vi "Cell Alignment to Horizontal and Vertical.vi"() -> ()   [LabVIEW 2019, in "Exaprom PDF.lvlib"]
doc: "Developed by Jean-Marc Simard\nCopyright © 2012, Exaprom Inc.\nAll rights reserved.\nLicense: BSD\n\nWith iTextSharp 4.1.6 (http://itextsharp.sourceforge.net)\nunder Mozilla Public License Version 1.1\n(http://www.mozilla.org/MPL/MPL-1.1.html)"
uses:
  Controls/Table Controls/Cell Alignment 20px.ctl
  Controls/Text Controls/Texte alignement.ctl
  Controls/Table Controls/Cell Vertical alignment.ctl
  Exaprom PDF.lvlib
panel:
  out "Vertical":T1=enum."MIDDLE"
  out "Horizontal":T2=enum."CENTER" caption="Align"
  in  "Cell Alignment":T3
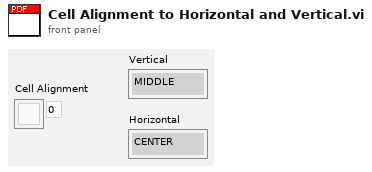
[diagram p1: front panel]
types:
  T1 = typedef "Exaprom PDF.lvlib/Cell Vertical alignment.ctl" = enum16{"TOP", "MIDDLE", "BOTTOM"}
  T2 = typedef "Exaprom PDF.lvlib/Texte alignement.ctl" = enum16{"Select", "CENTER", "JUSTIFY", "LEFT", "RIGHT"}
  T3 = typedef "Exaprom PDF.lvlib/Cell Alignment 20px.ctl" = u16
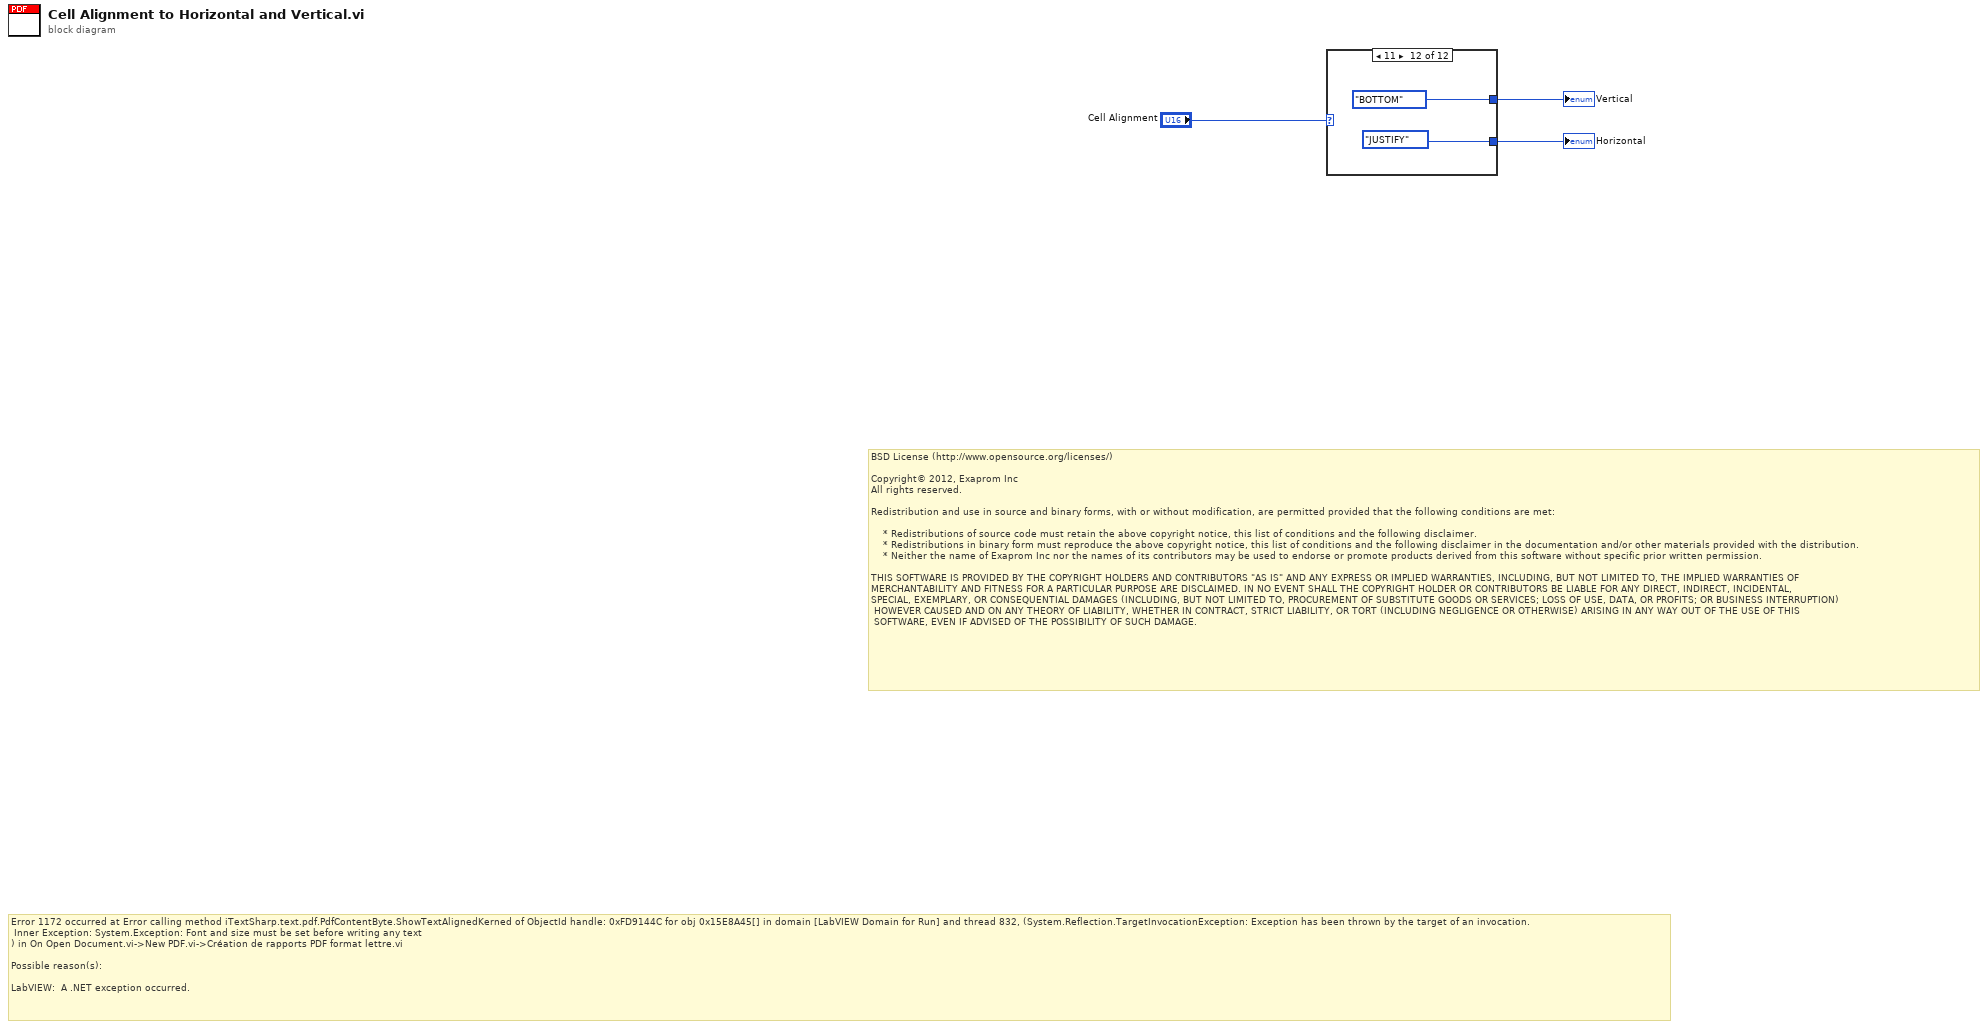
[diagram p0: block diagram]
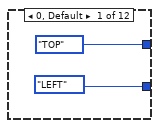
[diagram p2: hidden frame]
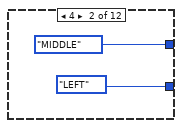
[diagram p3: hidden frame]
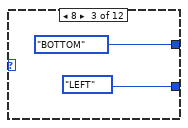
[diagram p4: hidden frame]
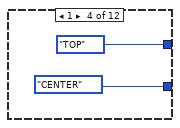
[diagram p5: hidden frame]
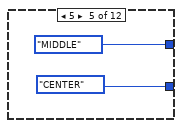
[diagram p6: hidden frame]
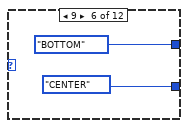
[diagram p7: hidden frame]
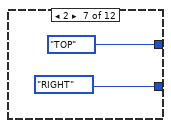
[diagram p8: hidden frame]
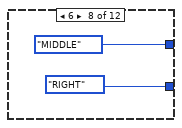
[diagram p9: hidden frame]
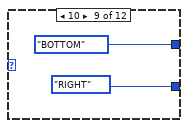
[diagram p10: hidden frame]
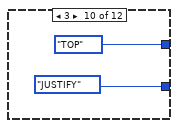
[diagram p11: hidden frame]
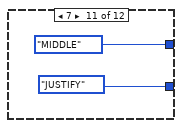
[diagram p12: hidden frame]
diagram:
  # "Error 1172 occurred at Error calling method iTextSharp.text.pdf.PdfContentByte.ShowTextAlignedKerned of ObjectId handle: 0xFD9144C for obj 0x15E8A45[] in domain [LabVIEW Domain for Run] and thread 832, (System.Reflection.TargetInvocationException: Exception has been thrown by the target of an invocation.\n\tInner Exception: System.Exception: Font and size must be set before writing any text\n) in On Open Document.vi->New PDF.vi->Création de rapports PDF format lettre.vi\n\nPossible reason(s):\n\nLabVIEW:  A .NET exception occurred."
  # "BSD License (http://www.opensource.org/licenses/)\n\nCopyright© 2012, Exaprom Inc\nAll rights reserved.\n\nRedistribution and use in source and binary forms, with or without modification, are permitted provided that the following conditions are met:\n\n    * Redistributions of source code must retain the above copyright notice, this list of conditions and the following disclaimer.\n    * Redistributions in binary form must reproduce the above copyright notice, this list of conditions and the following disclaimer in the documentation and/or other materials provided with the distribution.\n    * Neither the name of Exaprom Inc nor the names of its contributors may be used to endorse or promote products derived from this software without specific prior written permission.\n\nTHIS SOFTWARE IS PROVIDED BY THE COPYRIGHT HOLDERS AND CONTRIBUTORS \"AS IS\" AND ANY EXPRESS OR IMPLIED WARRANTIES, INCLUDING, BUT NOT LIMITED TO, THE IMPLIED WARRANTIES OF \nMERCHANTABILITY AND FITNESS FOR A PARTICULAR PURPOSE ARE DISCLAIMED. IN NO EVENT SHALL THE COPYRIGHT HOLDER OR CONTRIBUTORS BE LIABLE FOR ANY DIRECT, INDIRECT, INCIDENTAL,\nSPECIAL, EXEMPLARY, OR CONSEQUENTIAL DAMAGES (INCLUDING, BUT NOT LIMITED TO, PROCUREMENT OF SUBSTITUTE GOODS OR SERVICES; LOSS OF USE, DATA, OR PROFITS; OR BUSINESS INTERRUPTION)\n HOWEVER CAUSED AND ON ANY THEORY OF LIABILITY, WHETHER IN CONTRACT, STRICT LIABILITY, OR TORT (INCLUDING NEGLIGENCE OR OTHERWISE) ARISING IN ANY WAY OUT OF THE USE OF THIS\n SOFTWARE, EVEN IF ADVISED OF THE POSSIBILITY OF SUCH DAMAGE."
  n1 = case shown="11" "Cell Alignment" {
    tunnel: [Cell_Vertical_alignment."TOP" ("Vertical") Cell_Vertical_alignment."MIDDLE" ("Vertical") Cell_Vertical_alignment."BOTTOM" ("Vertical") Cell_Vertical_alignment."TOP" ("Vertical") Cell_Vertical_alignment."MIDDLE" ("Vertical") Cell_Vertical_alignment."BOTTOM" ("Vertical") Cell_Vertical_alignment."TOP" ("Vertical") Cell_Vertical_alignment."MIDDLE" ("Vertical") Cell_Vertical_alignment."BOTTOM" ("Vertical") Cell_Vertical_alignment."TOP" ("Vertical") Cell_Vertical_alignment."MIDDLE" ("Vertical") Cell_Vertical_alignment."BOTTOM" ("Vertical")] -> w2
    tunnel: [Texte_alignement."LEFT" ("Horizontal") Texte_alignement."LEFT" ("Horizontal") Texte_alignement."LEFT" ("Horizontal") Texte_alignement."CENTER" ("Horizontal") Texte_alignement."CENTER" ("Horizontal") Texte_alignement."CENTER" ("Horizontal") Texte_alignement."RIGHT" ("Horizontal") Texte_alignement."RIGHT" ("Horizontal") Texte_alignement."RIGHT" ("Horizontal") Texte_alignement."JUSTIFY" ("Horizontal") Texte_alignement."JUSTIFY" ("Horizontal") Texte_alignement."JUSTIFY" ("Horizontal")] -> w1
    frame 0, Default {
    }
    frame 4 {
    }
    frame 8 {
    }
    frame 1 {
    }
    frame 5 {
    }
    frame 9 {
    }
    frame 2 {
    }
    frame 6 {
    }
    frame 10 {
    }
    frame 3 {
    }
    frame 7 {
    }
    frame 11 {
    }
  }
  "Horizontal" <- w1
  "Vertical" <- w2
